vi "Initialize.vi"(7 "writer buffer size":i32, 8 "error in (no error)":errorcluster, 9 "reader url":string, 10 "writer name":string) -> (0 "error out":errorcluster, 3 "NetworkStreamWriter out":refnum<class "NetworkStreamWriter.lvclass">)   [LabVIEW 2011, in "NetworkStreamWriter.lvclass"]
doc: "This VI returns an instance of the NetworkStreamWriter class. A NetworkStreamWriter attempts to open a network stream with a reader endpoint. As with network streams, the writer url on the reader or the reader url on the writer must be given before the connection can be made. Note that until a connection is made, this VI will not return. It will, however, stop on a commanded e-stop from the top-level VI. This VI also launches a writer daemon which constantly sends information added to the internal queue by the Write method across the network stream."
uses:
  NetworkStreamWriter.lvclass
  NetworkStreamWriter.lvclass/NetworkStreamWriter.ctl
  WriterDaemon.vi
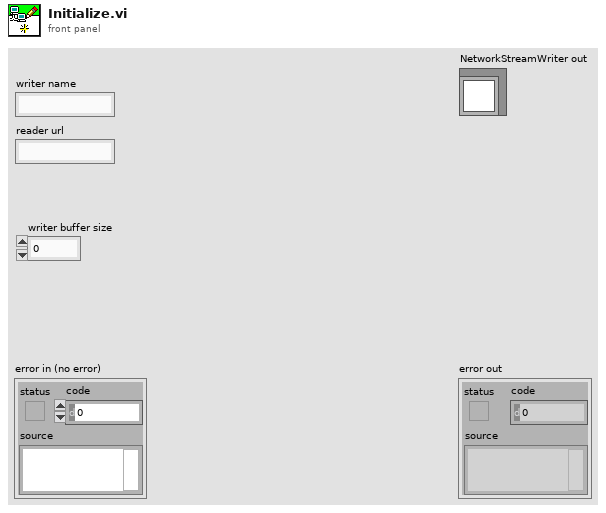
[diagram p1: front panel]
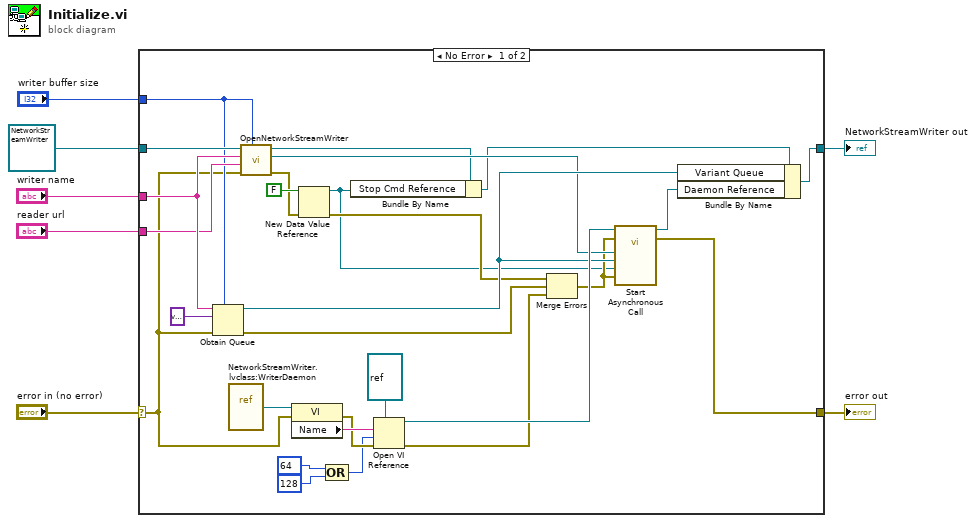
[diagram p0: block diagram]
diagram:
  n1 = case shown="No Error" "error in (no error)" {
    selector: "error in (no error)" -> [w25 w37]
    tunnel: [w19 w37] -> w6
    tunnel: [w30 w36] -> w5
    tunnel: refnum<class "NetworkStreamWriter.lvclass"> refnum ("NetworkStreamWriter in") -> [w35 w36]
    tunnel: "writer name" -> [w34 _]
    tunnel: "reader url" -> [w33 _]
    tunnel: "writer buffer size" -> [w31 _]
    frame No Error {
      n2 = Obtain Queue(max queue size (-1, unlimited)=w31, name (unnamed)=w34, element data type=variant, error in (no error)=w25) -> (queue out=w21:refnum<queue>, error out=w22:errorcluster)  [unwired: 1 in, 1 out]
      n3 = vi-ref "NetworkStreamWriter.lvclass:WriterDaemon.vi"() -> (w29:refnum<vi>)
      n4 = call "OpenNetworkStreamWriter.vi"("writer buffer size"=w31, "error in (no error)"=w25, "reader url"=w33, "writer name"=w34, "NetworkStreamWriter in"=w35) -> ("error out"=w12:errorcluster, "Writer Endpoint"=w20:refnum<k21>, "NetworkStreamWriter out"=w11:refnum<class "NetworkStreamWriter.lvclass">)  [unwired: 4 in]
      n5 = property class="VI"(reference=w29, error in=w25) -> (error out=w24:errorcluster, "Name"=w28:string)  [unwired: 1 out]
      n6 = New Data Value Reference(data value=FALSE, error in=w12) -> (data value reference=w8:refnum<data-value>, error out=w9:errorcluster)
      n7 = Compound Arithmetic op=OR(64 ("options"), 128 ("options")) -> (w14:i32)
      n8 = Bundle By Name(cluster=w11, "Stop Cmd Reference"=w8) -> (w10:refnum<class "NetworkStreamWriter.lvclass">)
      n9 = Open VI Reference(type specifier VI Refnum (for type only)=refnum<vi> refnum, vi path=w28, options=w14, error in (no error)=w24) -> (vi reference=w27:refnum<vi>, error out=w23:errorcluster)  [unwired: 2 in]
      n10 = Merge Errors(w9, w22, w23) -> (w18:errorcluster)
      n11 = call-by-ref "Start Asynchronous Call"(reference=w27, error in=w18, 8:"error in (no error)"=w18, "Stop Cmd Reference"=w8, "Variant Queue"=w21, "Writer Endpoint"=w20) -> (reference out=w17:refnum<vi>, error out=w19:errorcluster)  [unwired: 8 in]
      n12 = Bundle By Name(cluster=w10, "Variant Queue"=w21, "Daemon Reference"=w17) -> (w30:refnum<class "NetworkStreamWriter.lvclass">)
    }
    frame Error {
    }
  }
  "error out" <- w6
  "NetworkStreamWriter out" <- w5
